vi "InitLaser.vi"(7 "error in (no error)":errorcluster, 9 "remote port or service name":u16=50002, 10 "Laser IP Adress":string="192.168.0.11") -> (0 "error out":errorcluster={"status"=TRUE, "code"=54, "source"="TCP Open Connection in InitLaser.vi"}, 3 "connection ID":refnum<k5>)   [LabVIEW 2018]
doc: "Laser Init (Laser Initialization) makes the connection between Keyence laser and labview via TCP"
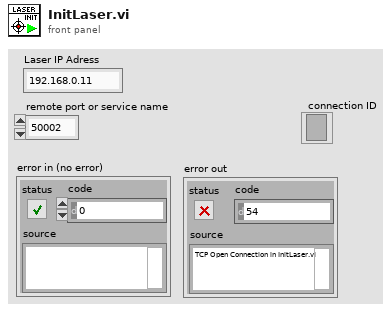
[diagram p1: front panel]
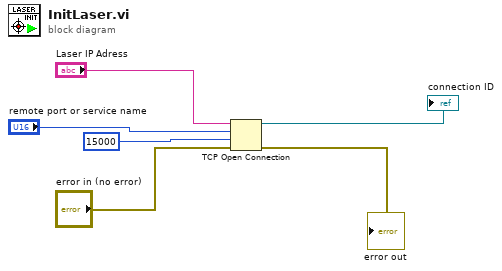
[diagram p0: block diagram]
diagram:
  n1 = TCP Open Connection(address="Laser IP Adress", remote port or service name="remote port or service name", timeout ms (60000)=15000, error in (no error)="error in (no error)") -> (connection ID=→"connection ID":refnum<k5>, error out=→"error out":errorcluster)  [unwired: 1 in]
